vi "test_2consecutiveLaunchShouldReturnError.vi"(11 "Test Case In":refnum<class "TaskControllerTests.lvclass">) -> (0 "error out":errorcluster, 3 "Test Case Out":refnum<class "TaskControllerTests.lvclass">)   [LabVIEW 2023, in "TaskControllerTests.lvclass"]
uses:
  TaskControllerTests.lvclass
  <vilib>/Astemes/LUnit/Test Case.lvclass/Test Case.ctl
  <vilib>/Astemes/LUnit/Palette/Pass If Error.vi
  <vilib>/Astemes/LUnit/Palette/Advanced Assertions/Pass If Specific Error.vi/d0e67a5c-31db-4060-a993-98defbf94426.vi
  <vilib>/Astemes/LUnit/Palette/Fail.vi
  <vilib>/Astemes/LUnit/Core/LUnit Test Case/Private/Append Fail Result.vi
  <vilib>/Astemes/LUnit/Core/LUnit Test Case/Private/Append Pass Result.vi
  <vilib>/Astemes/LUnit/Core/LUnit Test Case/Private/Run In UI.vi
  TaskMock/TaskMock.lvclass
  <vilib>/Comparison/Equal/Equal Functor/Equal Functor.lvclass
  TaskControllerTests.lvclass/TaskControllerTests.ctl
  source/TaskController/TaskController.lvclass
  <vilib>/Astemes/LUnit/Palette/Advanced Assertions/LUnit Advanced Assertions.lvlib
  C:/Program Files (x86)/National Instruments/LabVIEW 2023/vi.lib/Astemes/LUnit/Test Case.lvclass
  C:/Program Files (x86)/National Instruments/LabVIEW 2023/vi.lib/Astemes/LUnit/LUnit Runnable.lvclass
  C:/projects/TLC_Daemon/tests/TaskControllerTests/TaskControllerTests.lvclass
  C:/projects/TLC_Daemon/tests/TaskMock/TaskMock.lvclass
  C:/projects/TLC_Daemon/source/ITask/ITask.lvclass
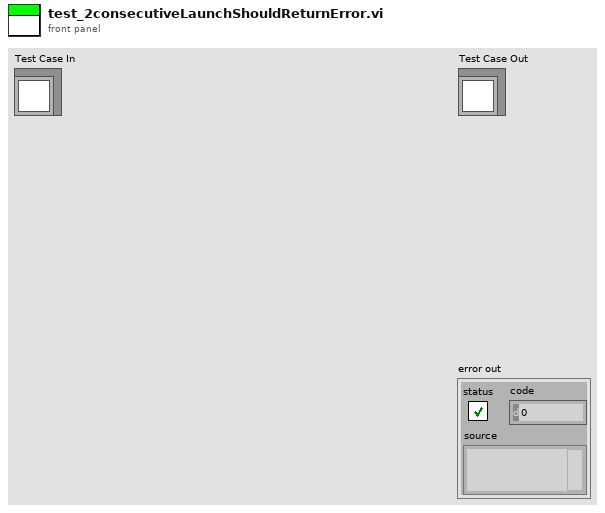
[diagram p1: front panel]
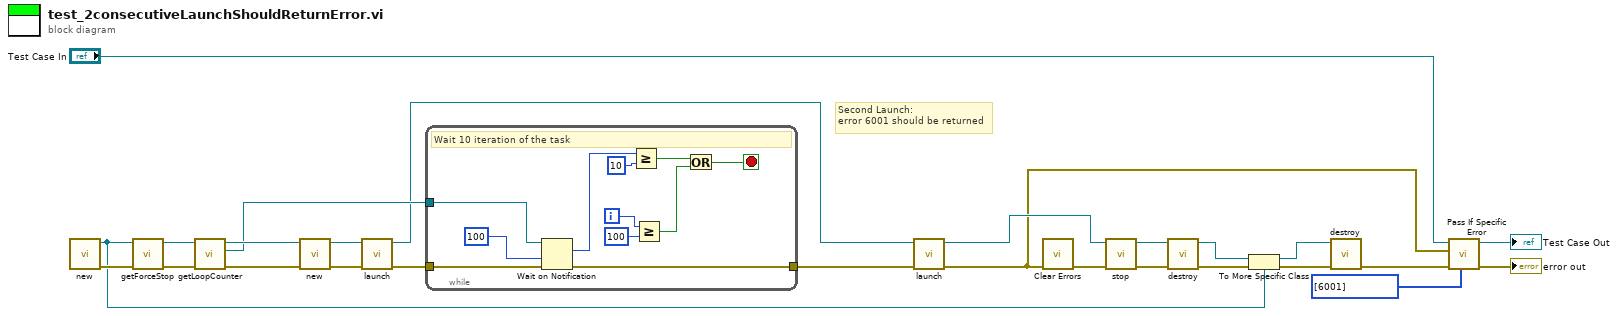
[diagram p0: block diagram]
diagram:
  # "Second Launch:\nerror 6001 should be returned"
  n1 = call "new.vi"() -> ("error out"=w17:errorcluster, "TaskMock out"=w12:refnum<class "TaskMock.lvclass">)  [unwired: 10 in]
  n2 = call "getForceStop.vi"("error in (no error)"=w17, "TaskMock in"=w12) -> ("error out"=w14:errorcluster, "TaskMock out"=w13:refnum<class "TaskMock.lvclass">)  [unwired: 7 in, 1 out]
  n3 = call "getLoopCounter.vi"("error in (no error)"=w14, "TaskMock in"=w13) -> ("error out"=w16:errorcluster, "loopCounter"=w10:refnum<notifier>, "TaskMock out"=w20:refnum<class "TaskMock.lvclass">)  [unwired: 7 in]
  n4 = call "new.vi"("error in (no error)"=w16, "task"=w20) -> ("error out"=w22:errorcluster, "TaskController out"=w23:refnum<class "TaskController.lvclass">)  [unwired: 8 in]
  n5 = call "launch.vi"("error in (no error)"=w22, "TaskController in"=w23) -> ("error out"=w21:errorcluster, "TaskController out"=w7:refnum<class "TaskController.lvclass">)  [unwired: 8 in]
  n6 = while {
    tunnel: w21 -> [w28]
    tunnel: w10 -> [w37]
    tunnel: [w27] -> w8
    i -> [w33]
    stop <- w30 stop-if-true
    # "Wait 10 iteration of the task"
    n7 = Wait on Notification(notifier=w37, timeout in ms (-1)=100, error in (no error)=w28) -> (notification=w35:i32, error out=w27:errorcluster)  [unwired: 1 in, 2 out]
    n8 = Greater Or Equal?(x=w35, y=10) -> (x >= y?=w31:bool)
    n9 = Greater Or Equal?(x=w33, y=100) -> (x >= y?=w29:bool)
    n10 = Or(x=w31, y=w29) -> (x .or. y?=w30:bool)
  }
  n11 = call "launch.vi"("error in (no error)"=w8, "TaskController in"=w7) -> ("error out"=w4:errorcluster, "TaskController out"=w6:refnum<class "TaskController.lvclass">)  [unwired: 8 in]
  n12 = call <vilib>:"Clear Errors.vi"("error in (no error)"=w4) -> ("error out"=w3:errorcluster)  [unwired: 5 in, 1 out]
  n13 = call "stop.vi"("error in (no error)"=w3, "TaskController in"=w6) -> ("error out"=w5:errorcluster, "TaskController out"=w15:refnum<class "TaskController.lvclass">)  [unwired: 8 in]
  n14 = call "destroy.vi"("error in (no error)"=w5, "TaskController in"=w15) -> ("error out"=w2:errorcluster, "taskResult"=w19:refnum<class "ITask.lvclass">)  [unwired: 8 in]
  n15 = To More Specific Class(target class=w12, reference=w19, error in=w2) -> (specific class reference=w18:refnum<class "TaskMock.lvclass">, error out=w1:errorcluster)
  n16 = call "destroy.vi"("error in (no error)"=w1, "TaskMock in"=w18) -> ("error out"=w9:errorcluster)  [unwired: 9 in]
  n17 = call <vilib>:"Pass If Specific Error.vi"("Error Codes"=i32[] [6001], "error in (no error)"=w9, "Assert error"=w4, "LUnit Test Case In"="Test Case In") -> ("error out"=→"error out":errorcluster, "LUnit Test Case Out"=→"Test Case Out":refnum<class "TaskControllerTests.lvclass">)  [unwired: 6 in]
